vi "Read ID-attribute.vi"(8 "error in (no error)":errorcluster, 11 "ID in":refnum<class "ID.lvclass">) -> (0 "error out":errorcluster, 2 "ID-attribute":T1, 3 "ID out":refnum<class "ID.lvclass">)   [LabVIEW 2013, in "MaterialCharacterization.lvlib" / "ID.lvclass"]
uses:
  ID.lvclass
  Attribute-ID.ctl
  ID.lvclass/ID.ctl
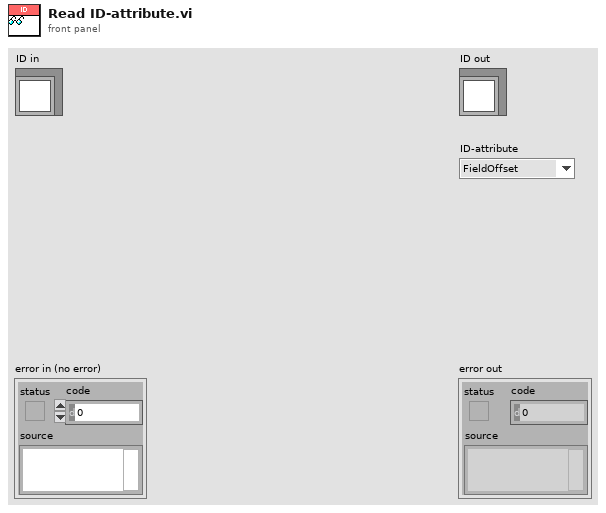
[diagram p1: front panel]
types:
  T1 = typedef "MaterialCharacterization.lvlib/ID.lvclass/Attribute-ID.ctl" = enum16{"FieldOffset", "TransformEnable", "Transform", "Units", "XYCalFactor", "EnableLaser", "JumpDelay", "MarkDelay", "PolyDelay", "LaserOnDelay", "LaserOffDelay", "JumpSpeed", "MarkSpeed", "LaserPowerDelay", "LaserEnableDelay", "LaserPower", "Offset"}
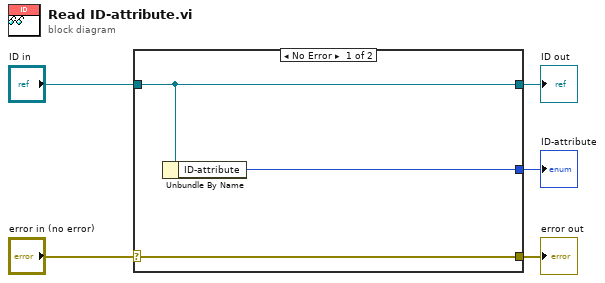
[diagram p0: block diagram]
diagram:
  n1 = case shown="No Error" "error in (no error)" {
    selector: "error in (no error)" -> [w8 w9]
    tunnel: [w8 w9] -> w4
    tunnel: [w7 w10] -> w2
    tunnel: "ID in" -> [w7 w10]
    tunnel: [w6 _] -> w1
    frame No Error {
      n2 = Unbundle By Name(w7) -> ("ID-attribute"=w6:T1)
    }
    frame Error {
    }
  }
  "error out" <- w4
  "ID out" <- w2
  "ID-attribute" <- w1
